vi "Open Front Panel.vi"(8 "error in (no error)":errorcluster, 11 "Measure Object in":refnum<class "Template Module.lvclass">) -> (0 "error out":errorcluster, 3 "Measure Object out":refnum<class "Template Module.lvclass">)   [LabVIEW 2016, in "Template Module.lvclass"]
uses:
  Template Module.lvclass
  Template Module.lvclass/Template Module.ctl
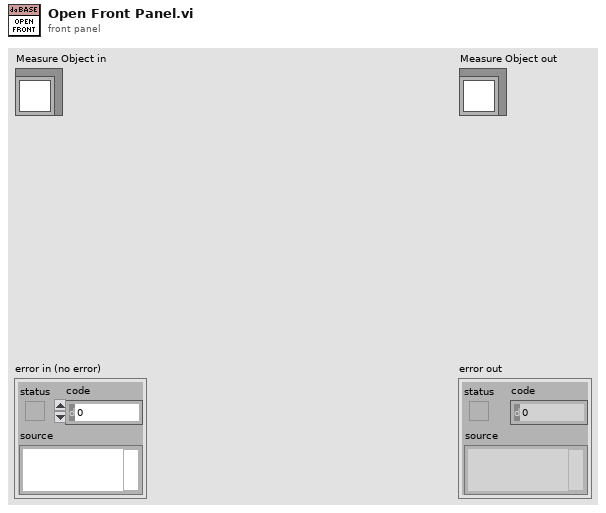
[diagram p1: front panel]
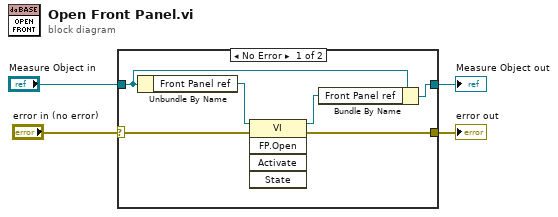
[diagram p0: block diagram]
diagram:
  n1 = case shown="No Error" "error in (no error)" {
    selector: "error in (no error)" -> [w10 w12]
    tunnel: [w9 w12] -> w3
    tunnel: [w6 w11] -> w1
    tunnel: "Measure Object in" -> [w8 w11]
    frame No Error {
      n2 = Unbundle By Name(w8) -> ("Front Panel ref"=w7:refnum<vi>)
      n3 = invoke class="VI" method="FP.Open"(reference=w7, error in=w10) -> (reference out=w5:refnum<vi>, error out=w9:errorcluster)  [unwired: 3 in, 3 out]
      n4 = Bundle By Name(cluster=w8, "Front Panel ref"=w5) -> (w6:refnum<class "Template Module.lvclass">)
    }
    frame Error {
    }
  }
  "error out" <- w3
  "Measure Object out" <- w1
